vi "Read TDM Channel Groups.vi"() -> ()   [LabVIEW 2023]
doc: "Reads channel groups from a TDM file."
uses:
  <vilib>/Platform/storage/lvStorage.llb/_openFunction.ctl
  <vilib>/Platform/storage/lvStorage.llb/_openStorageWithRootAutoDetect.vi
  <vilib>/Platform/storage/lvStorage.llb/xStorage/xStorageSupp/ErrorOut.vi
  <vilib>/Platform/storage/Storage.llb/__loadPropRefList.vi
  <vilib>/Platform/storage/Storage.llb/__loadPropString.vi
  <vilib>/Platform/storage/Storage.llb/__loadPropTime.vi
  <vilib>/Platform/storage/lvStorage.llb/_loadDDT.vi
  <vilib>/Platform/storage/Storage.llb/Get Object Info.vi
  <vilib>/Platform/storage/Storage.llb/__closeStorageFromObject.vi
  <vilib>/Platform/storage/lvStorage.llb/xStorage/Open Data Storage/Open Data Storage.xnode
  <vilib>/Platform/storage/lvStorage.llb/xStorage/Get Properties/Get Properties.xnode
  <vilib>/Platform/storage/lvStorage.llb/xStorage/Close Data Storage/Close Data Storage.xnode
panel:
  out "Channel Group Names":string[](array[string])
  out "Time Stamp":timestamp
  out "Title":string
  out "Name":string
  out "Channel Data from File":dynamicdata(graph)
  # "Overview: Demonstrates the use of the DataPlugin Express VIs to read channel group data from a TDM file.\nRequirements: Windows\nInstructions:\n1. Make sure you have already run Write TDM Channel Groups.vi.\n2. Run this VI. The contents of the TDM file will be displayed below.\n3. Delete the TDM file (located at [LabVIEW Data]\\Example Channel Group File.tdm) when you are done."
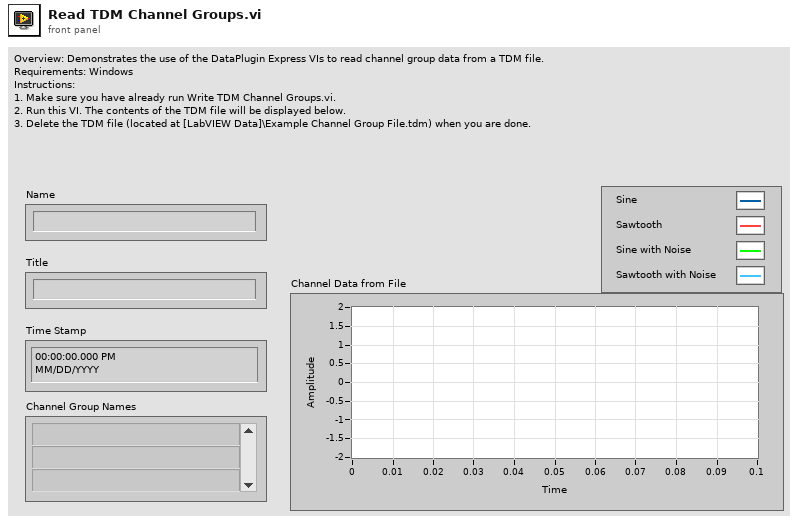
[diagram p1: front panel]
types:
  T1 = enum16{"UPDATE", "READ", "QUERY", "CREATE CHILD", "CREATE", "CONNECT", "DISCONNECT"}
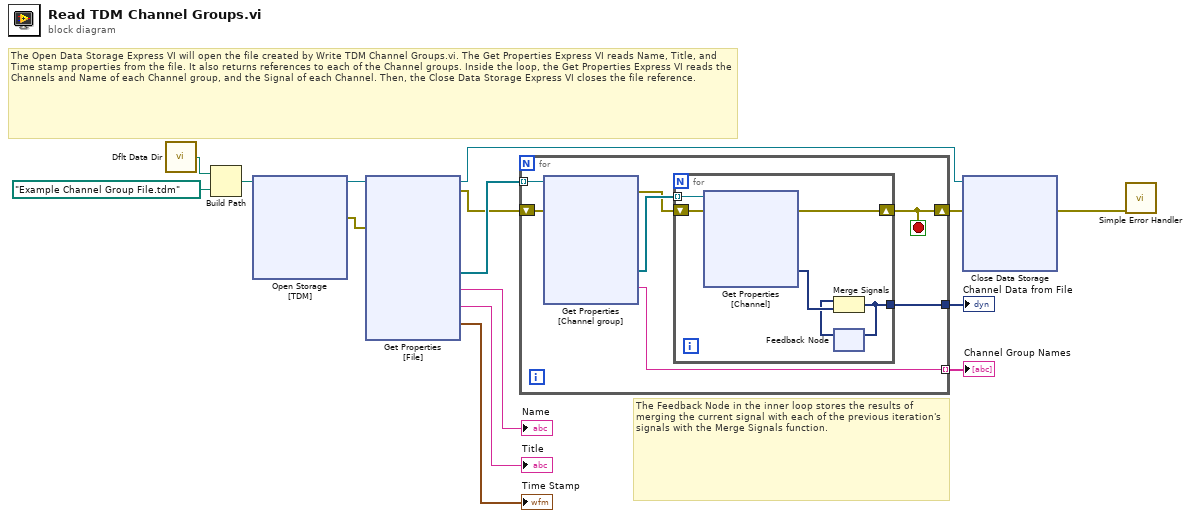
[diagram p0: block diagram]
diagram:
  # "The Feedback Node in the inner loop stores the results of merging the current signal with each of the previous iteration's signals with the Merge Signals function."
  # "The Open Data Storage Express VI will open the file created by Write TDM Channel Groups.vi. The Get Properties Express VI reads Name, Title, and Time stamp properties from the file. It also returns references to each of the Channel groups. Inside the loop, the Get Properties Express VI reads the Channels and Name of each Channel group, and the Signal of each Channel. Then, the Close Data Storage Express VI closes the file reference."
  n1 = call <vilib>:"Dflt Data Dir.vi"() -> ("App:Default Data Directory"=w10:path)
  n2 = Build Path(base path=w10, name or relative path=path "Example Channel Group File.tdm" ("default name")) -> (appended path=w8:path)
  n3 = xnode "Open Storage\n[TDM]"("file path"=w8) -> ("storage refnum (file)"=w15:refnum<k20>, "error out"=w14:errorcluster)  [unwired: 2 in, 3 out]
  n4 = xnode "Get Properties\n[File]"("storage refnum (file)"=w15, "error in"=w14) -> ("storage refnums (channel group)"=w13:refnum<k20>[], "Name"=→"Name":string, "Title"=→"Title":string, "Time stamp"=→"Time Stamp":timestamp, "storage refnum (file) out"=w7:refnum<k20>, "error out"=w12:errorcluster)
  n5 = for {
    tunnel: w13 -> [w22] mode=indexing
    shift-right: [w16] -> w11
    shift-left: w12 -> [w21]
    tunnel: [w19] -> w6
    tunnel: [w17] -> w2 mode=indexing
    stop <- w16 stop-if-true
    n6 = xnode "Get Properties\n[Channel group]"("storage refnum (channel group)"=w22, "error in"=w21) -> ("storage refnums (channel)"=w20:refnum<k20>[], "Name"=w17:string, "error out"=w18:errorcluster)  [unwired: 1 out]
    n7 = for {
      tunnel: w20 -> [w40] mode=indexing
      shift-right: [w38] -> w16
      shift-left: w18 -> [w39]
      tunnel: [w35] -> w19
      n8 = xnode "Get Properties\n[Channel]"("storage refnum (channel)"=w40, "error in"=w39) -> ("Signal"=w37:dynamicdata, "error out"=w38:errorcluster)  [unwired: 2 out]
      n9 = feedback #1() -> (w36:dynamicdata)  [unwired: 1 in]
      n10 = Merge Signals(w36, w37) -> (w35:dynamicdata)
      n11 = feedback-in #1(w35) -> ()
    }
  }
  "Channel Data from File" <- w6
  "Channel Group Names" <- w2
  n12 = xnode "Close Data Storage\n"("storage refnum (file)"=w7, "error in (no error)"=w11) -> ("error out"=w1:errorcluster)  [unwired: 1 out]
  n13 = call <vilib>:"Simple Error Handler.vi"("error in (no error)"=w1) -> ()  [unwired: 1 in, 8 out]
